vi "test_AlarmLogging.vi"   [LabVIEW 2009]
uses:
  controls/sec_AlarmStates_enum.ctl
  modules/alarm logging/sec_Log_Command_enum.ctl
types:
  T1 = typedef "sec_Log_Command_enum.ctl" = enum16{"Initialise", "Log Alarms"}
  T2 = typedef "sec_AlarmStates_enum.ctl" = enum16{"Normal", "Alarm", "Bypass", "Tamper"}
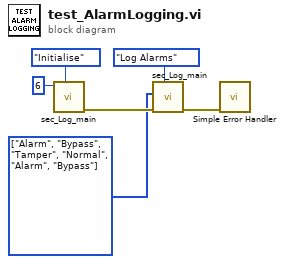
[diagram p0: block diagram]
diagram:
  w3 = T2[] [enum."Alarm", enum."Bypass", enum."Tamper", enum."Normal", enum."Alarm", enum."Bypass"] items=["Normal", "Alarm", "Bypass", "Tamper"] ("Alarm States")
  n1 = call "sec_Log_main.vi"("Command"=sec_Log_Command_enum."Initialise", "Number Of Alarms"=6) -> ("error out"=w4:errorcluster)  [unwired: 9 in]
  n2 = call "sec_Log_main.vi"("Command"=sec_Log_Command_enum."Log Alarms", "error in (no error)"=w4, "Alarm States"=w3) -> ("error out"=w1:errorcluster)  [unwired: 8 in]
  n3 = call <vilib>:"Simple Error Handler.vi"("error in (no error)"=w1) -> ()  [unwired: 4 in, 5 out]
